vi "DeadBand.vi"(8 "Error In":errorcluster, 9 "Threshold":dbl, 10 "Process Variable":dbl, 11 "Send Value":dbl) -> (0 "Error Out":errorcluster, 3 "Output":dbl)   [LabVIEW 2016]
doc: "Send Value - The Value to Output when Below Threshold\nProcess Variable - Input to Dead Band subVI, will use Absolute Value\nThreshold - Value to Exceed"
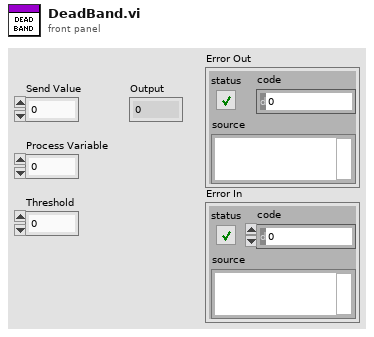
[diagram p1: front panel]
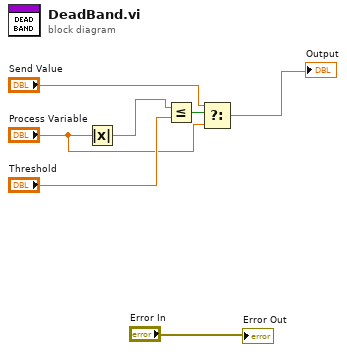
[diagram p0: block diagram]
diagram:
  n1 = Absolute Value(x="Process Variable") -> (abs(x)=w2:dbl)
  n2 = Less Or Equal?(x=w2, y="Threshold") -> (x <= y?=w5:bool)
  n3 = Select(t="Send Value", s=w5, f="Process Variable") -> (s? t:f=→"Output":dbl)
  "Error Out" <- "Error In"
